vi "Configure Current Max.vi"(8 "error in (no error)":errorcluster, 10 "Set Current Max (0 A)":dbl format="%.2f", 11 "VISA resource name":refnum<visa-resource-name>) -> (0 "error out":errorcluster, 3 "VISA resource name out":refnum<visa-resource-name>)   [LabVIEW 2021, in "Sorensen M9A Series.lvlib"]
doc: "This VI sets the upper soft limit for output current for the Sorensen power supply. If the soft limit is exceeded, or if the soft limit value is lower than then present output current setting, the power supply will ignore the command, turn on the ERR LED, and set the ERR bit in the Status and Serial Poll Registers. Units are in Amps."
uses:
  Sorensen M9A Series.lvlib
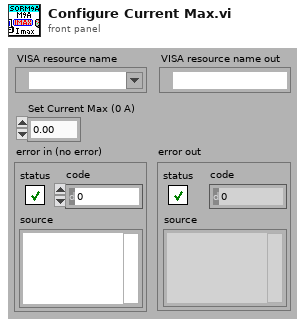
[diagram p1: front panel]
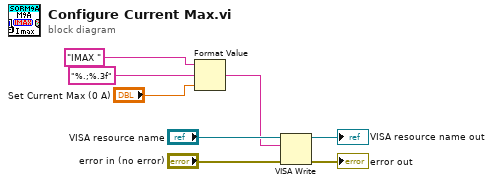
[diagram p0: block diagram]
diagram:
  n1 = Format Value(string ("")="IMAX " ("data"), format string="%.;%.3f", value (0)="Set Current Max (0 A)") -> (output string=w4:string)
  n2 = VISA Write(VISA resource name="VISA resource name", write buffer=w4, error in (no error)="error in (no error)") -> (VISA resource name out=→"VISA resource name out":refnum<visa-resource-name>, error out=→"error out":errorcluster)  [unwired: 1 out]
